vi "main.vi"() -> ()   [LabVIEW 2020]
panel:
  in  "STOP":bool
  in  "Tab Control":enum32{"RUN", "Config"}(tab)
  in  "rbox_no":string(combo) caption="box number"
  in  "cbox_no":string(combo) caption="box number"
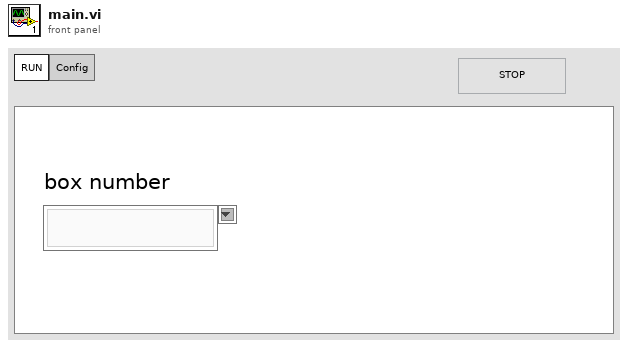
[diagram p1: front panel]
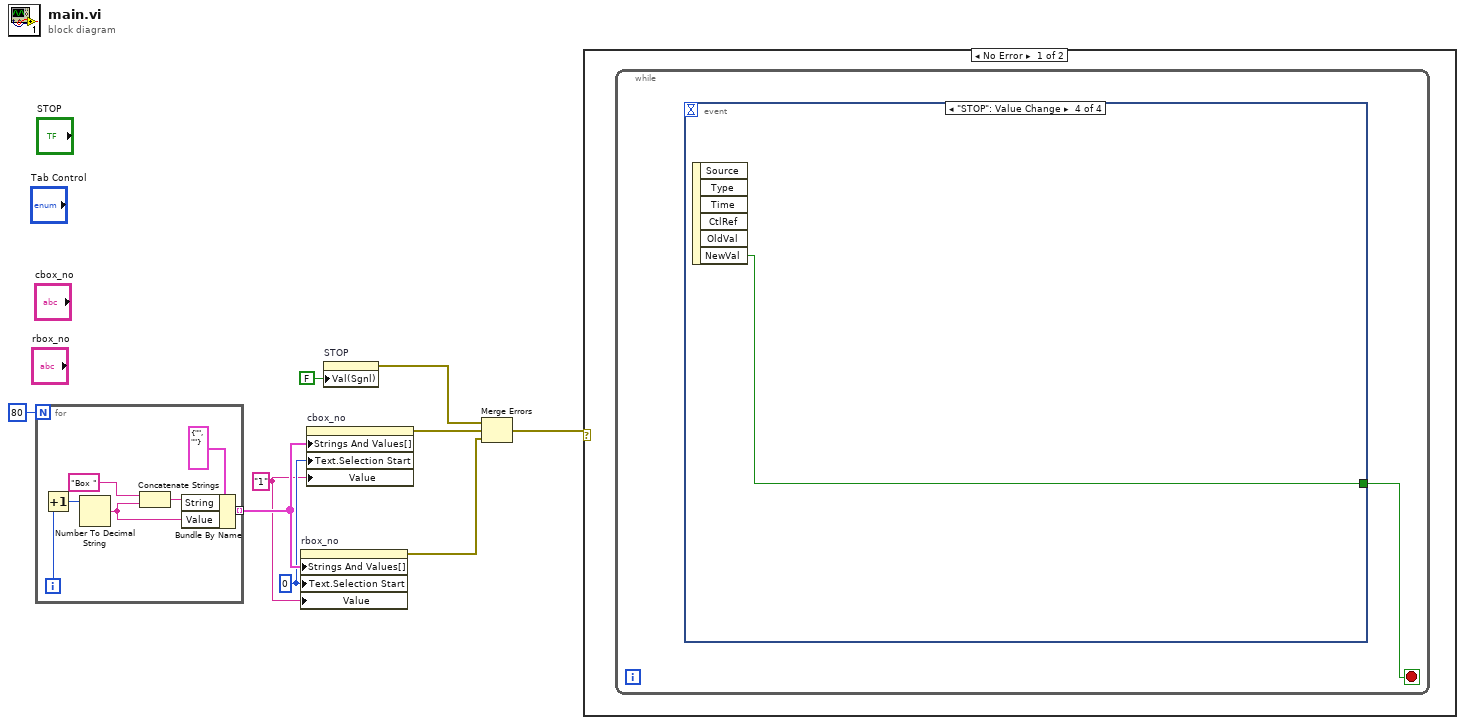
[diagram p0: block diagram]
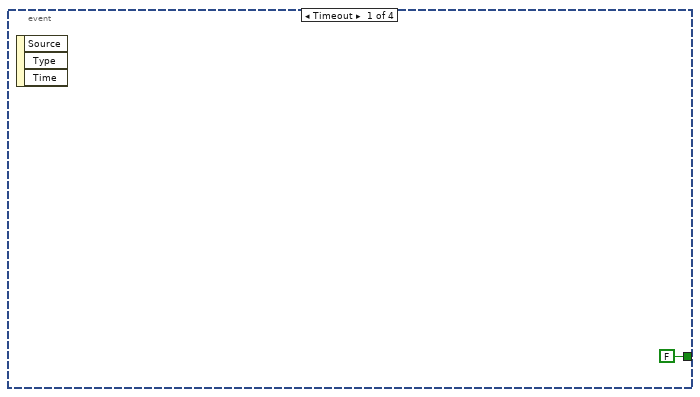
[diagram p2: hidden frame]
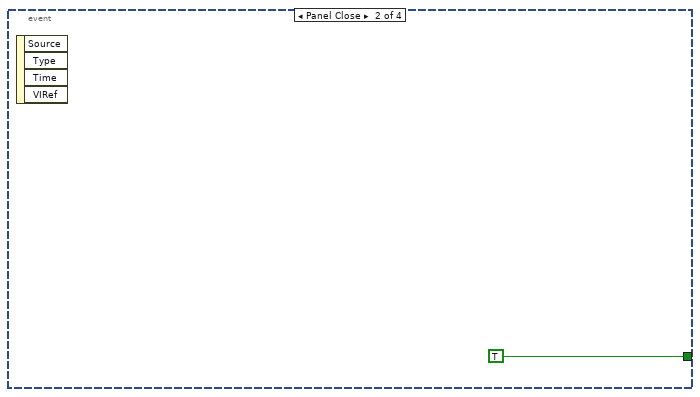
[diagram p3: hidden frame]
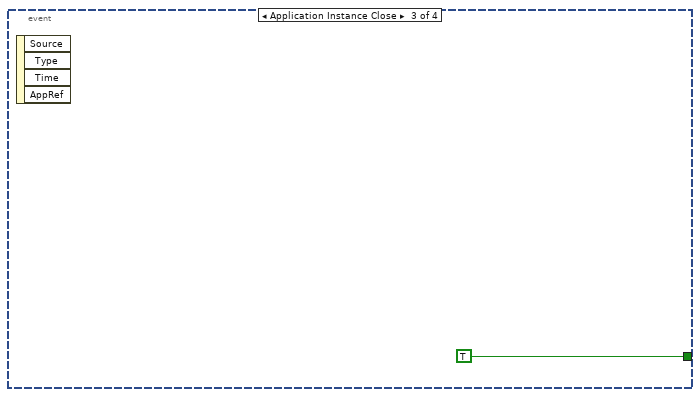
[diagram p4: hidden frame]
diagram:
  w6 = "1"
  w7 = u32 0 ("Text.Selection:Start")
  n1 = for {
    N: 80 -> [_]
    tunnel: [w14] -> w8 mode=indexing
    i -> [w16]
    n2 = Increment(x=w16) -> (x+1=w15:i32)
    n3 = Number To Decimal String(number=w15) -> (decimal integer string=w11:string)  [unwired: 1 in]
    n4 = Concatenate Strings("Box " ("string"), w11) -> (w12:string)
    n5 = Bundle By Name(cluster=cluster{"String":string, "Value":string} {"String"="", "Value"=""} ("input cluster"), "String"=w12, "Value"=w11) -> (w14:cluster{"String":string, "Value":string})
  }
  n6 = property on="rbox_no" class="CmbBox"("Strings And Values[]"=w8, "Text.Selection Start"=w7, "Value"=w6) -> (error out=w4:errorcluster)  [unwired: 2 in, 1 out]
  n7 = property on="cbox_no" class="CmbBox"("Strings And Values[]"=w8, "Text.Selection Start"=w7, "Value"=w6) -> (error out=w5:errorcluster)  [unwired: 2 in, 1 out]
  n8 = property on="STOP" class="Bool (strict)"("Val(Sgnl)"=FALSE ("Value (Signaling)")) -> (error out=w2:errorcluster)  [unwired: 2 in, 1 out]
  n9 = Merge Errors(w2, w5, w4) -> (w3:errorcluster)
  n10 = case shown="No Error" w3 {
    frame No Error {
      n11 = while {
        stop <- w17 stop-if-true
        n12 = event shown="[3] \"STOP\": Value Change" {
          selector: _ -> [_ _ _ _]
          dyn-events: _ -> [_ _ _ _]
          timeout: _ -> [_ _ _ _]
          tunnel: [FALSE TRUE TRUE w21] -> w17
          event Timeout {
            n13 = event-data() -> ()  [unwired: 1 in, 3 out]
          }
          event Panel Close {
            n14 = event-data() -> ()  [unwired: 1 in, 4 out]
          }
          event Application Instance Close {
            n15 = event-data() -> ()  [unwired: 1 in, 4 out]
          }
          event "STOP": Value Change {
            n16 = event-data() -> ("NewVal"=w21:bool)  [unwired: 1 in, 5 out]
          }
        }
      }
    }
    frame Error {
    }
  }
